vi "Get Data.vi"(8 "error in (no error)":errorcluster, 11 "DataGrid.lvlib:Abstract EVENT.lvclass":refnum<class "Abstract EVENT.lvclass">) -> (0 "error out":errorcluster, 1 "Context":i32=1, 2 "ColumnIndex":i32, 3 "RowIndex":i32, 5 "Exception":refnum<k24>)   [LabVIEW 2016, in "DataGrid.lvlib" / "DataError.lvclass"]
uses:
  <userlib>/LabVIEWdotNetDataGrid/source/Events/DataError/DataError.lvclass
  <userlib>/LabVIEWdotNetDataGrid/source/Events/Abstract EVENT/Abstract EVENT.lvclass
  <userlib>/LabVIEWdotNetDataGrid/source/Events/DataError/DataError.lvclass/DataError.ctl
  <userlib>/LabVIEWdotNetDataGrid/source/Events/DataError/Read ColumnIndex.vi
  <userlib>/LabVIEWdotNetDataGrid/source/Events/DataError/Read Context.vi
  <userlib>/LabVIEWdotNetDataGrid/source/Events/DataError/Read Exception.vi
  <userlib>/LabVIEWdotNetDataGrid/source/Events/DataError/Read RowIndex.vi
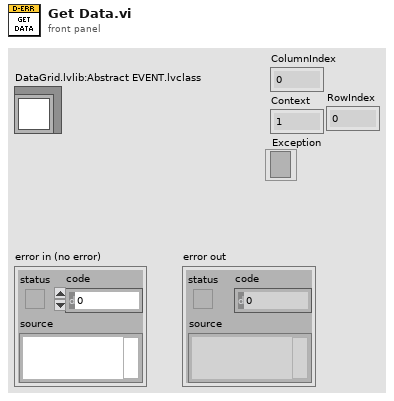
[diagram p1: front panel]
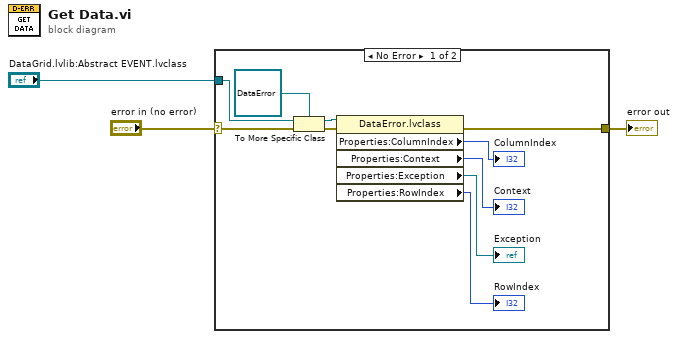
[diagram p0: block diagram]
diagram:
  n1 = case shown="No Error" "error in (no error)" {
    selector: "error in (no error)" -> [w10 w14]
    tunnel: [w13 w14] -> w2
    tunnel: "DataGrid.lvlib:Abstract EVENT.lvclass" -> [w12 _]
    frame No Error {
      n2 = To More Specific Class(target class=refnum<class "DataError.lvclass"> refnum ("DataGrid.lvlib:DataError.lvclass"), reference=w12, error in=w10) -> (specific class reference=w11:refnum<class "DataError.lvclass">, error out=w9:errorcluster)
      n3 = property class="DataError.lvclass"(reference=w11, error in=w9) -> (error out=w13:errorcluster, "Properties:ColumnIndex"=→"ColumnIndex":i32, "Properties:Context"=→"Context":i32, "Properties:Exception"=→"Exception":refnum<k24>, "Properties:RowIndex"=→"RowIndex":i32)  [unwired: 1 out]
    }
    frame Error {
    }
  }
  "error out" <- w2
